vi "main.vi"() -> ()   [LabVIEW 2015, in "lv-hello-world.lvlib"]
uses:
  lv-hello-world.lvlib
  <userlib>/antonio-alexander/lv-bin-windows/public/api/v1/v1.lvlib
panel:
  out "admin?":bool
  out "commit_hash":string
  out "version":string
  out "application_directory":path
  out "arguments":string[](array[string])
  in  "stop":bool
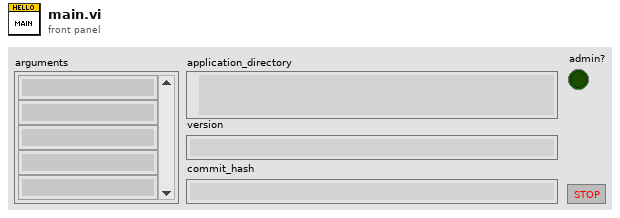
[diagram p1: front panel]
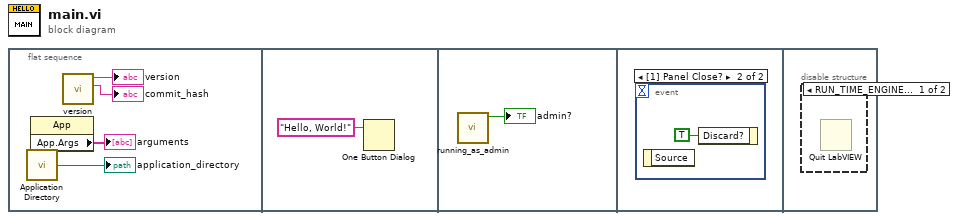
[diagram p0: block diagram]
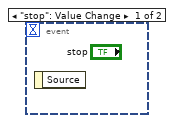
[diagram p2: hidden frame]
diagram:
  n1 = flat-sequence {
    frame #0 {
      n2 = call <vilib>:"Application Directory.vi"() -> ("Application Directory"=→"application_directory":path)
      n3 = property class="App"() -> ("App.Args"=→"arguments":string[])  [unwired: 2 in, 2 out]
      n4 = call "version.vi"() -> ("commit"=→"commit_hash":string, "version"=→"version":string)  [unwired: 8 in, 2 out]
    }
    frame #1 {
      n5 = One Button Dialog(message="Hello, World!") -> ()  [unwired: 1 in, 1 out]
    }
    frame #2 {
      n6 = call <userlib>:"running_as_admin.vi"() -> ("admin"=→"admin?":bool)  [unwired: 10 in, 1 out]
    }
    frame #3 {
      n7 = event shown="[1] Panel Close?" {
        selector: _ -> [_ _]
        dyn-events: _ -> [_ _]
        timeout: _ -> [_ _]
        event "stop": Value Change {
          n8 = event-data() -> ()  [unwired: 1 in, 1 out]
        }
        event Panel Close? {
          n9 = event-data() -> ()  [unwired: 1 in, 1 out]
          n10 = event-data("Discard?"=TRUE) -> ()  [unwired: 1 in, 1 out]
        }
      }
    }
    frame #4 {
      n11 = disable-structure shown="RUN_TIME_ENGINE==True" {
        frame condition #0 {
          n12 = Quit LabVIEW() -> ()  [unwired: 1 in]
        }
        frame condition #1 (active) {
        }
      }
    }
  }
